vi "Count Zero LSBs.vi"(0 "input":u32, 11 "error in (no error)":errorcluster) -> (4 "trailing zeros":i32, 15 "error out":errorcluster)   [LabVIEW 2020, in "NI_FpgaMspHost.lvlib"]
doc: "Returns the number of zeros on the right (LSB) side of a 32-bit integer input. If the input is equal to zero, <B>trailing zeros</B> returns zero."
uses:
  <vilib>/rvi/Analysis/host/Public/NI_FpgaMspHost.lvlib
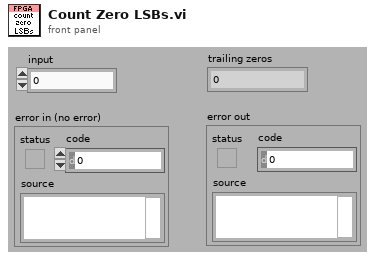
[diagram p1: front panel]
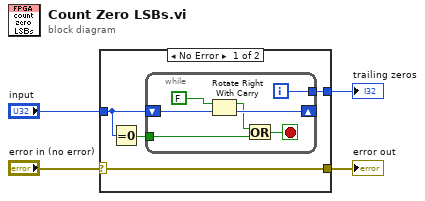
[diagram p0: block diagram]
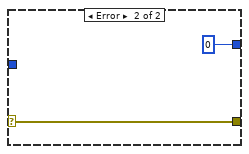
[diagram p2: hidden frame]
diagram:
  n1 = case shown="No Error" "error in (no error)" {
    selector: "error in (no error)" -> [w5 w17]
    tunnel: "input" -> [w8 _]
    tunnel: [w6 0] -> w3
    tunnel: [w5 w17] -> w1
    frame No Error {
      n2 = Equal To 0?(x=w8) -> (x = 0?=w7:bool)
      n3 = while {
        tunnel: w7 -> [w14]
        shift-right: [w11] -> _
        shift-left: w8 -> [w12]
        tunnel: [w9] -> w6
        i -> [w9]
        stop <- w13 stop-if-true
        n4 = Rotate Right With Carry(2:w12, 3:FALSE ("carry")) -> (0:w11:u32, 1:w10:bool)
        n5 = Or(x=w10, y=w14) -> (x .or. y?=w13:bool)
      }
    }
    frame Error {
    }
  }
  "trailing zeros" <- w3
  "error out" <- w1
